vi "SortChannels.vi"(0 "DisplayTetrodes in":refnum<class "DisplayTetrodes.lvclass">, 11 "error in (no error)":errorcluster) -> (1 "sortedTetChanNum":i32[](array[numeric]), 3 "sortedTetNum":i32[](array[numeric]), 4 "DisplayTetrodes out":refnum<class "DisplayTetrodes.lvclass">, 6 "reorderedChanNums":i32[](array[numeric]), 10 "sortedChanIdx":i32[](array[numeric]), 12 "unsortedTetNums":i32[](array[numeric]), 13 "reorderedDiodeChan":i32, 15 "error out":errorcluster)   [LabVIEW 2011, in "DisplayTetrodes.lvclass"]
uses:
  DisplayTetrodes.lvclass
  <vilib>/imath/engines/lvmath2/RunTimeEngine/ErrorHandling/NIMS_Finalize Error.vi
  <vilib>/imath/engines/lvmath2/RunTimeEngine/NodeEndStatement/NIMS_NodeEndStatement_Output.vi
  <instcachedir>/0/NIMS_NodeEndStatement_Output_53EC0D466D134D7ABD903AC30B43404B.lvgen/NIMS_NodeEndStatement_Output_53EC0D466D134D7ABD903AC30B43404B_004.vi
  <instcachedir>/0/NIMS_NodeEndStatement_Output_53EC0D466D134D7ABD903AC30B43404B.lvgen/NIMS_NodeEndStatement_Output_53EC0D466D134D7ABD903AC30B43404B_005.vi
  <instcachedir>/0/NIMS_NodeEndStatement_Output_53EC0D466D134D7ABD903AC30B43404B.lvgen/NIMS_NodeEndStatement_Output_53EC0D466D134D7ABD903AC30B43404B_001.vi
  <vilib>/imath/engines/lvmath2/RunTimeEngine/VariableToken/Read/NIMS_Get Elements - RV(_) - Check(_).vi
  <instcachedir>/0/NIMS_Get Elements - RV(_) - Check(_)_95E78A4FFA0646428F3543E57837F638.lvgen/NIMS_Get Elements - RV(_) - Check(_)_95E78A4FFA0646428F3543E57837F638_000.vi
  <vilib>/imathl/engines/lvmath/Functions/Error Handling/Create Error.vi
  <vilib>/imath/engines/lvmath2/RunTimeEngine/BuiltInFunctions/sort/NIMS_[2o]_sort(RRowV,I32,Str).vi
  <instcachedir>/0/NIMS_[2o]_sort(RRowV,I32,Str)_9DDE7701AB6E47E8854B392C2556FB2D.lvgen/NIMS_[2o]_sort(RRowV,I32,Str)_9DDE7701AB6E47E8854B392C2556FB2D_001.vi
  <vilib>/imath/engines/lvmath2/RunTimeEngine/VariableToken/Read/NIMS_Get Elements - RV(_) - Check.vi
  <instcachedir>/0/NIMS_Get Elements - RV(_) - Check_B511B9D8E05044FE80F9F088FE24B20C.lvgen/NIMS_Get Elements - RV(_) - Check_B511B9D8E05044FE80F9F088FE24B20C_003.vi
  <vilib>/imath/engines/lvmath2/RunTimeEngine/BuiltInFunctions/length/NIMS_length(GV).vi
  <instcachedir>/0/NIMS_length(GV)_08A3D13377FD4E4B96F5795FBF3698FA.lvgen/NIMS_length(GV)_08A3D13377FD4E4B96F5795FBF3698FA_002.vi
  <vilib>/imath/engines/lvmath2/RunTimeEngine/ReplaceToken/NIMS_Replace - Check Linear.vi
  <instcachedir>/0/NIMS_Replace - Check Linear_276AD648BD064726893CCF9ED6E2A728.lvgen/NIMS_Replace - Check Linear_276AD648BD064726893CCF9ED6E2A728_006.vi
  <vilib>/imath/engines/lvmath2/RunTimeEngine/RangeToken/NIMS_Range.vi
  <instcachedir>/0/NIMS_Range_0B7635FB69F84E19AA68E7FF959DF37C.lvgen/NIMS_Range_0B7635FB69F84E19AA68E7FF959DF37C_000.vi
  <vilib>/imath/engines/lvmath2/RunTimeEngine/ReplaceToken/NIMS_Replace - Size Check _(_)=VorM.vi
  <instcachedir>/0/NIMS_Replace - Size Check _(_)=VorM_C85DCC3888F14C5FACDCACC8CAF67F25.lvgen/NIMS_Replace - Size Check _(_)=VorM_C85DCC3888F14C5FACDCACC8CAF67F25_010.vi
  <vilib>/imath/engines/lvmath2/RunTimeEngine/ReplaceToken/NIMS_Replace - Assignment Check _(_)=VorM.vi
  <instcachedir>/0/NIMS_Replace - Assignment Check _(_)=VorM_486412C526DE41D4B9BEEA980C633181.lvgen/NIMS_Replace - Assignment Check _(_)=VorM_486412C526DE41D4B9BEEA980C633181_010.vi
  <vilib>/imath/engines/lvmath2/RunTimeEngine/ErrorHandling/NIMS_Create Error From Enums.vi
  <vilib>/imath/engines/lvmath2/RunTimeEngine/BuiltInFunctions/findnz/NIMS_[1o]_findnz(GRowV).vi
  <instcachedir>/0/NIMS_[1o]_findnz(GRowV)_FA69E315D4054D06B60D6FF1496271F7.lvgen/NIMS_[1o]_findnz(GRowV)_FA69E315D4054D06B60D6FF1496271F7_000.vi
  <vilib>/imath/engines/lvmath2/RunTimeEngine/BuiltInFunctions/is_empty/NIMS_is_empty(GV).vi
  <instcachedir>/0/NIMS_is_empty(GV)_FC7E7C3D9544432CB6AA2416ADCF6D56.lvgen/NIMS_is_empty(GV)_FC7E7C3D9544432CB6AA2416ADCF6D56_000.vi
  <vilib>/regexp/Match Regular Expression.xnode
panel:
  out "size(s) 2":i32
  out "size(s)":i32
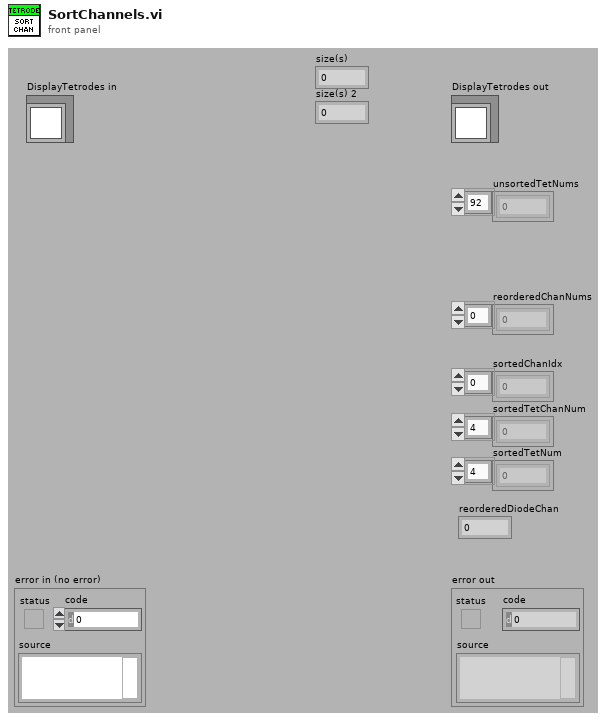
[diagram p1: front panel]
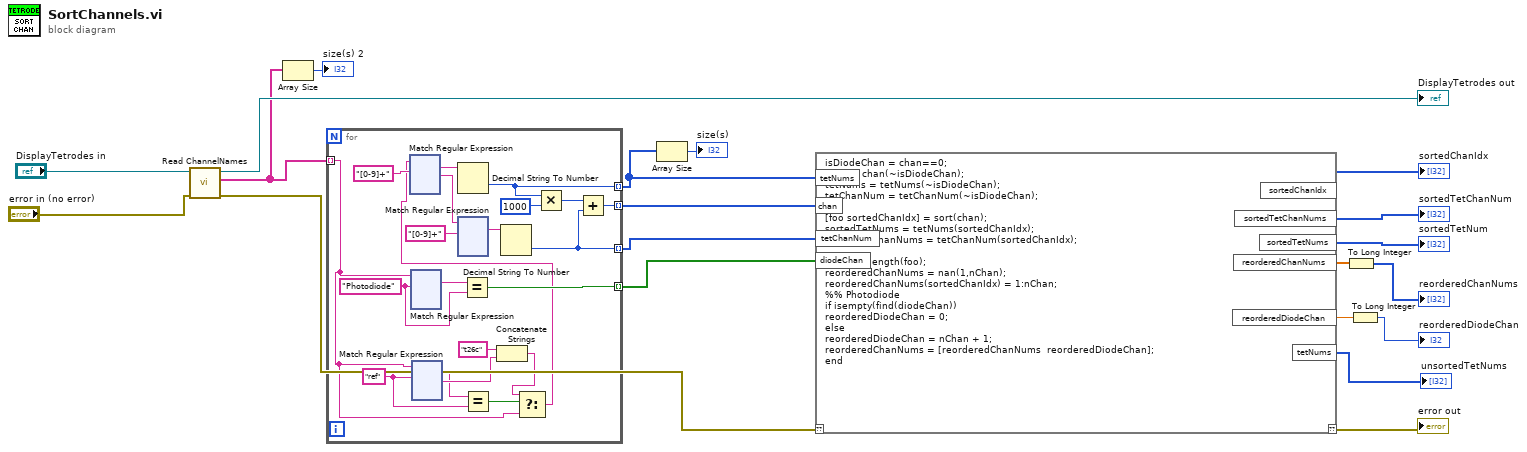
[diagram p0: block diagram]
diagram:
  n1 = call-dynamic "Read ChannelNames.vi"("error in (no error)"="error in (no error)", "DataReceiver in"="DisplayTetrodes in") -> ("error out"=w10:errorcluster, "ChannelNames"=w3:string[], "DataReceiver out"=→"DisplayTetrodes out":refnum<class "DisplayTetrodes.lvclass">)  [unwired: 7 in]
  n2 = Array Size(array=w3) -> (size(s)=→"size(s) 2":i32)
  n3 = for {
    tunnel: w3 -> [w22] mode=indexing
    tunnel: [w30] -> w19 mode=indexing
    tunnel: [w34] -> w5 mode=indexing
    tunnel: [w33] -> w20 mode=indexing
    tunnel: [w29] -> w8 mode=indexing
    w25 = "ref" ("regular expression")
    w31 = "Photodiode" ("regular expression")
    n4 = xnode "Match Regular Expression"("input string"=w22, "regular expression"=w31) -> ("whole match"=w32:string)  [unwired: 4 in, 4 out]
    n5 = xnode "Match Regular Expression"("input string"=w22, "regular expression"=w25) -> ("whole match"=w26:string, "after match"=w27:string)  [unwired: 4 in, 3 out]
    n6 = Equal?(x=w32, y=w31) -> (x = y?=w29:bool)
    n7 = Equal?(x=w26, y=w25) -> (x = y?=w24:bool)
    n8 = Concatenate Strings("t26c" ("string"), w27) -> (w23:string)
    n9 = Select(t=w23, s=w24, f=w22) -> (s? t:f=w21:string)
    n10 = xnode "Match Regular Expression"("input string"=w21, "regular expression"="[0-9]+") -> ("whole match"=w38:string, "after match"=w39:string)  [unwired: 4 in, 3 out]
    n11 = Decimal String To Number(string=w38) -> (number=w34:i32)  [unwired: 2 in, 1 out]
    n12 = xnode "Match Regular Expression"("input string"=w39, "regular expression"="[0-9]+") -> ("whole match"=w37:string)  [unwired: 4 in, 4 out]
    n13 = Decimal String To Number(string=w37) -> (number=w33:i32)  [unwired: 2 in, 1 out]
    n14 = Multiply(x=w34, y=1000) -> (x*y=w35:i32)
    n15 = Add(x=w35, y=w33) -> (x+y=w30:i32)
  }
  n16 = Array Size(array=w5) -> (size(s)=→"size(s)":i32)
  n17 = mathscript code="isDiodeChan = chan==0;\nchan = chan(~isDiodeChan);\ntetNums = tetNums(~isDiodeChan);\ntetChanNum = tetChanNum(~isDiodeChan);\n\n[foo sortedChanIdx] = sort(chan);\nsortedTetNums = tetNums(sortedChanIdx);\nsortedTetChanNums = tetChanNum(sortedChanIdx);\n\nnChan = length(foo);\nreorderedChanNums = nan(1,nChan);\nreorderedChanNums(sortedChanIdx) = 1:nChan;\n%% Photodiode\nif isempty(find(diodeChan))\nreorderedDiodeChan = 0;\nelse\nreorderedDiodeChan = nChan + 1;\nreorderedChanNums = [reorderedChanNums  reorderedDiodeChan];\nend"("??"=w10, "chan"=w19, "tetNums"=w5, "tetChanNum"=w20, "diodeChan"=w8) -> ("??"=→"error out":errorcluster, "sortedTetChanNums"=→"sortedTetChanNum":i32[], "sortedTetNums"=→"sortedTetNum":i32[], "sortedChanIdx"=→"sortedChanIdx":i32[], "reorderedChanNums"=w15:dbl[], "reorderedDiodeChan"=w7:dbl, "tetNums"=→"unsortedTetNums":i32[])
  n18 = To Long Integer(number=w15) -> (32bit integer=→"reorderedChanNums":i32[])
  n19 = To Long Integer(number=w7) -> (32bit integer=→"reorderedDiodeChan":i32)
